vi "Close.vi"(8 "error in (no error)":errorcluster, 11 "FPGA_Concrete in":refnum<class "FPGA_Concrete.lvclass">) -> (0 "error out":errorcluster, 3 "FPGA_Concrete out":refnum<class "FPGA_Concrete.lvclass">)   [LabVIEW 2019, in "FPGA_Concrete.lvclass"]
uses:
  FPGA_Concrete.lvclass
  FPGA_Concrete.lvclass/FPGA_Concrete.ctl
  <vilib>/FPGAPlugInAG/Dynamic/niLvFpga_Close_Dynamic.vi
  <vilib>/rvi/interface/nirviCloseFPGA/nirviCloseFPGA.xnode
  FPGA VI Reference.ctl
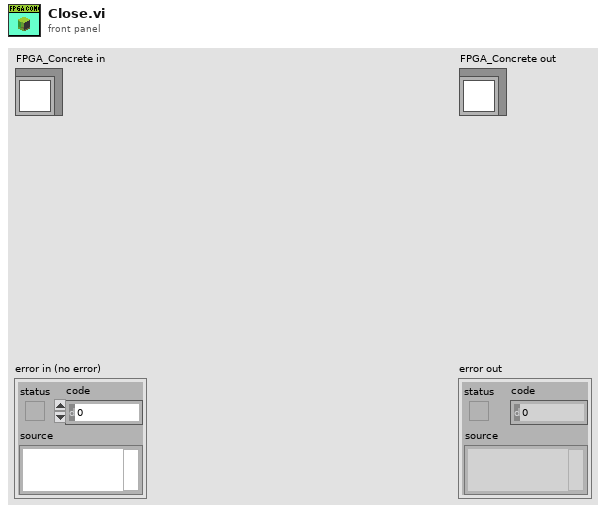
[diagram p1: front panel]
types:
  T1 = typedef "FPGA_Concrete.lvclass/FPGA VI Reference.ctl" = refnum<k20>
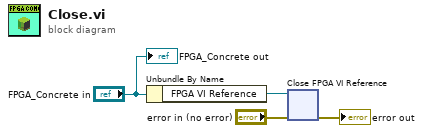
[diagram p0: block diagram]
diagram:
  n1 = Unbundle By Name("FPGA_Concrete in") -> ("FPGA VI Reference"=w3:T1)
  n2 = xnode "Close FPGA VI Reference"("FPGA VI Reference In"=w3, "error in"="error in (no error)") -> ("error out"=→"error out":errorcluster)
  "FPGA_Concrete out" <- "FPGA_Concrete in"
